vi "Page_Source_Pre_Add.vi"(6 "bottomTree?":bool, 8 "error in (no error)":errorcluster, 10 "AB_Source in":refnum<class "AB_Source.lvclass">, 11 "AB_PackedLibrary in":refnum<class "AB_PackedLibrary.lvclass">) -> (0 "error out":errorcluster, 2 "AB_Source out":refnum<class "AB_Source.lvclass">, 3 "AB_PackedLibrary out":refnum<class "AB_PackedLibrary.lvclass">)   [LabVIEW 2020, in "AB_PackedLibrary.lvclass"]
uses:
  <vilib>/AppBuilder/AB_Classes/PackedLib/AB_PackedLibrary.lvclass
  <vilib>/AppBuilder/AB_Classes/Source/AB_Source.lvclass
  <vilib>/AppBuilder/AB_Classes/Source/Library/AB_Source_Library.lvclass
  e:/builds/penguin/labview/branches/2020/dev/dist/vi.lib/AppBuilder/AB_Classes/Source/AB_Source.lvclass
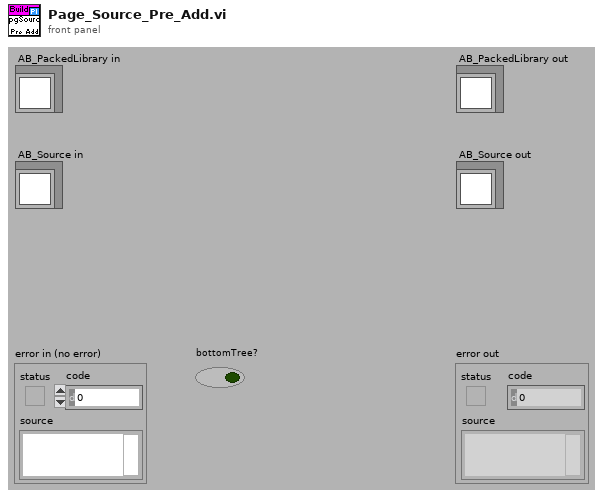
[diagram p1: front panel]
types:
  T1 = typedef "AB_Source.ctl" = cluster{"path":path, "itemID":string, "parentIndex":i32, "sourceInclusion":T2, "destinationIndex":i32, "properties":T3[], "newName":string, "lvfile":bool, "valid":bool, "eng_inBuild":bool, "eng_isNonVILink":bool, "Amalgamation":bool, "Amalgamation Piece":bool, "eng_delimitedName":string, "preventRename":bool}
  T2 = typedef "AB_Source_Inclusion.ctl" = enum16{"IncludeIfReferenced", "Include", "Exclude", "TopLevel"}
  T3 = typedef "AB_Source_Properties.ctl" = cluster{"sourcePropertyType":T4, "value":variant}
  T4 = typedef "AB_Source_Property_Type.ctl" = enum16{"Remove block diagram", "Remove front panel", "Password", "Window has title bar", "Show menu bar", "Show vertical scroll bar", "Show horizontal scroll bar", "Show toolbar", "Show Abort button", "Show fp when called", "Window behavior", "Allow user to close window", "Window run-time position", "Run when opened", "Allow debugging", "Auto error handling", "Generate guard code", "Use stack variables", "Expression folding", "Integer only", "Inline subVI"}
  T5 = typedef "AB_Source_Library.ctl" = cluster{"relinkCallers":bool, "atomicCopy":bool, "allowMissingMembers":bool, "eng_newDelimitedName":string, "eng_hasNonVILinks":bool, "eng_reference":refnum<vi>, "LVLIBPtopLevel":bool}
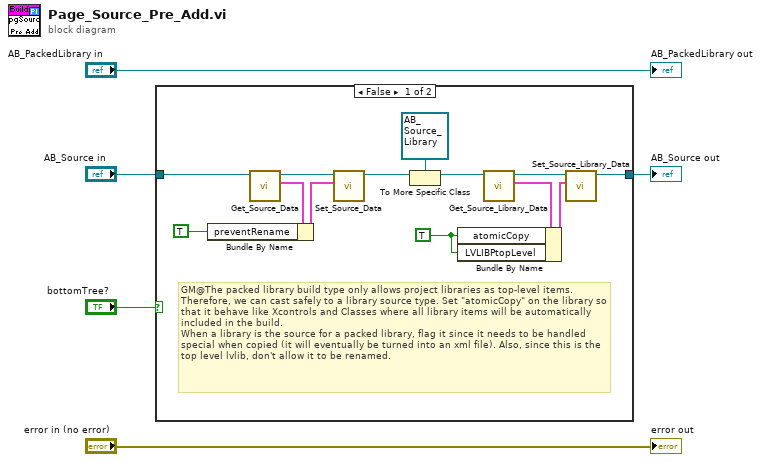
[diagram p0: block diagram]
diagram:
  n1 = case shown="False" "bottomTree?" {
    tunnel: [w13 w19] -> w3
    tunnel: "AB_Source in" -> [w10 w19]
    frame False {
      w12 = TRUE ("atomicCopy")
      # "GM@The packed library build type only allows project libraries as top-level items. Therefore, we can cast safely to a library source type. Set \"atomicCopy\" on the library so that it behave like Xcontrols and Classes where all library items will be automatically included in the build.\nWhen a library is the source for a packed library, flag it since it needs to be handled special when copied (it will eventually be turned into an xml file). Also, since this is the top level lvlib, don't allow it to be renamed."
      n2 = call <vilib>:"Get_Source_Data.vi"("Class in"=w10) -> ("data"=w8:T1, "Class out"=w11:refnum<class "AB_Source.lvclass">)  [unwired: 8 in, 1 out]
      n3 = Bundle By Name(cluster=w8, "preventRename"=TRUE) -> (w7:T1)
      n4 = call <vilib>:"Set_Source_Data.vi"("data"=w7, "Class in"=w11) -> ("Class out"=w9:refnum<class "AB_Source.lvclass">)  [unwired: 8 in, 1 out]
      n5 = To More Specific Class(target class=refnum<class "AB_Source_Library.lvclass"> refnum ("AB_Source_Library.lvclass"), reference=w9) -> (specific class reference=w17:refnum<class "AB_Source_Library.lvclass">)  [unwired: 1 in, 1 out]
      n6 = call <vilib>:"Get_Source_Library_Data.vi"("Class in"=w17) -> ("data"=w14:T5, "Class out"=w16:refnum<class "AB_Source_Library.lvclass">)  [unwired: 8 in, 1 out]
      n7 = Bundle By Name(cluster=w14, "atomicCopy"=w12, "LVLIBPtopLevel"=w12) -> (w15:T5)
      n8 = call <vilib>:"Set_Source_Library_Data.vi"("data"=w15, "Class in"=w16) -> ("Class out"=w13:refnum<class "AB_Source_Library.lvclass">)  [unwired: 8 in, 1 out]
    }
    frame True {
      # "If adding to bottom tree there is no need to modify the source item."
    }
  }
  "AB_Source out" <- w3
  "error out" <- "error in (no error)"
  "AB_PackedLibrary out" <- "AB_PackedLibrary in"
